vi "4.6.3.vi"() -> ()   [LabVIEW 2017]
panel:
  in  "stop":bool
  in  "b":dbl
  out "和":dbl
  in  "a":dbl
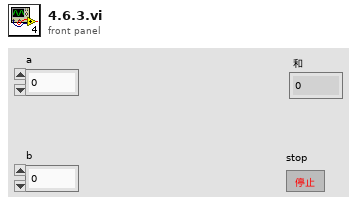
[diagram p1: front panel]
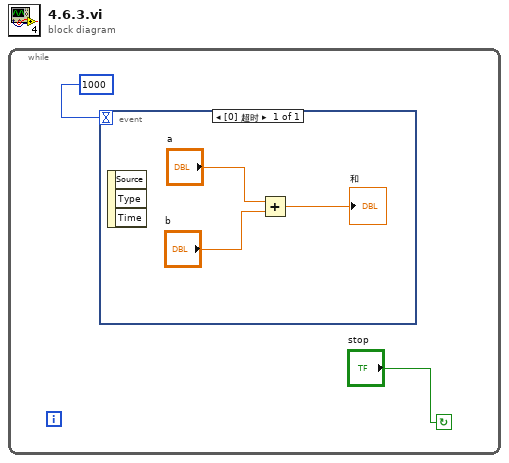
[diagram p0: block diagram]
diagram:
  n1 = while {
    stop <- "stop" continue-if-true
    n2 = event shown="[0] 超时" {
      selector: _ -> [_]
      dyn-events: _ -> [_]
      timeout: 1000 -> [_]
      event Timeout {
        n3 = event-data() -> ()  [unwired: 1 in, 3 out]
        n4 = Add(x="a", y="b") -> (x+y=→"和":dbl)
      }
    }
  }
